vi "Ping Address.vi"(8 "error in (no error)":errorcluster, 9 "Number of pings(4)":i32=4, 10 "IP Address(loopback=127.0.0.1)":string="127.0.0.1", 11 "object in":refnum<class "Ghetto_ping.lvclass">) -> (0 "error out":errorcluster, 1 "Valid network address?":bool, 2 "Ping output":string, 3 "object out":refnum<class "Ghetto_ping.lvclass">)   [LabVIEW 2013, in "Ghetto_ping.lvclass"]
uses:
  Ghetto_ping.lvclass
panel:
  # "I AM REENTRANT"
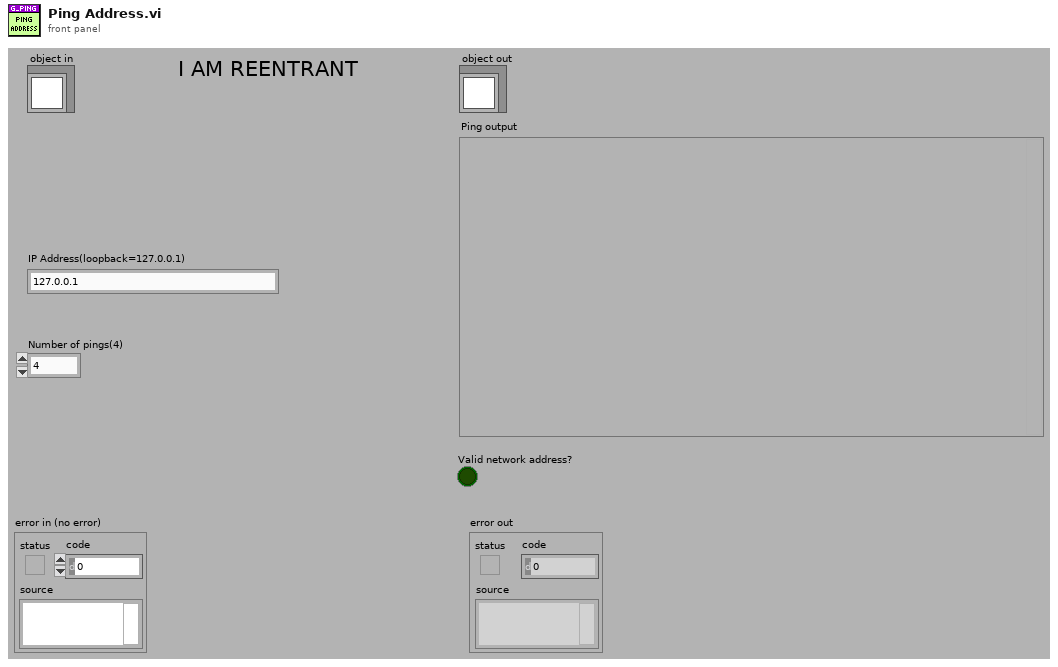
[diagram p1: front panel]
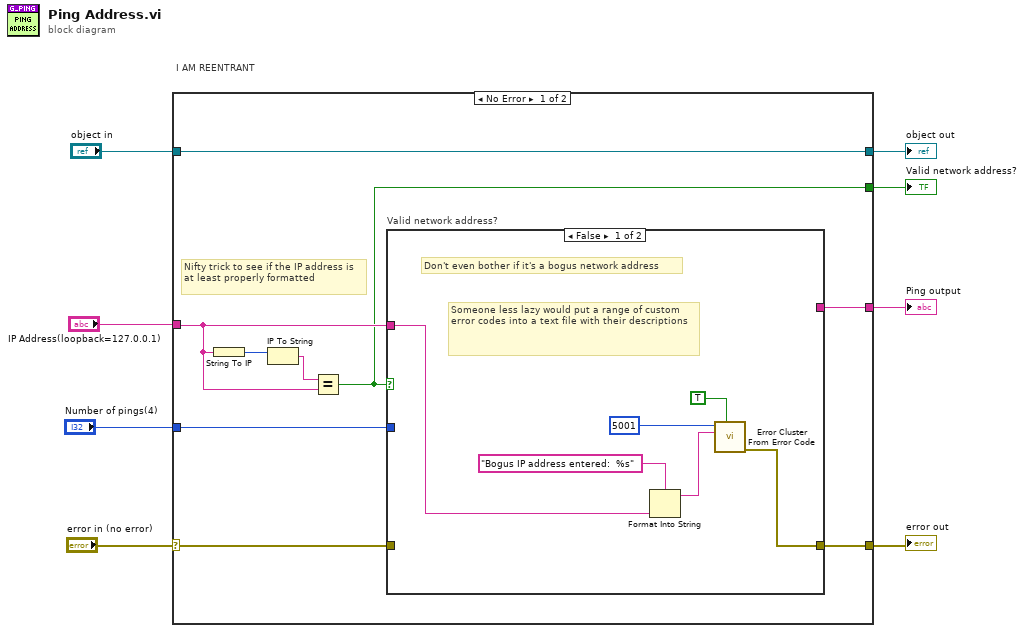
[diagram p0: block diagram]
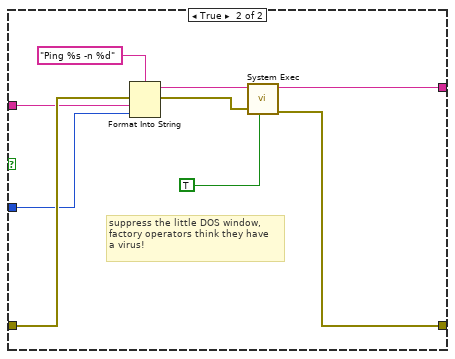
[diagram p2: hidden frame]
diagram:
  # "I AM REENTRANT"
  n1 = case shown="No Error" "error in (no error)" {
    selector: "error in (no error)" -> [w16 w34]
    tunnel: [w15 w34] -> w7
    tunnel: [w17 w33] -> w5
    tunnel: "object in" -> [w17 w33]
    tunnel: "IP Address(loopback=127.0.0.1)" -> [w10 _]
    tunnel: [w14 _] -> w3
    tunnel: "Number of pings(4)" -> [w13 _]
    tunnel: [w9 _] -> w1
    frame No Error {
      # "Nifty trick to see if the IP address is at least properly formatted"
      n2 = String To IP(1:w10) -> (0:w12:u32)
      n3 = IP To String(2:w12) -> (0:w11:string)  [unwired: 1 in]
      n4 = Equal?(x=w11, y=w10) -> (x = y?=w9:bool)
      n5 = case "Valid network address?" shown="False" w9 {
        tunnel: w16 -> [_ w28]
        tunnel: [w18 w27] -> w15
        tunnel: [_ w26] -> w14
        tunnel: w13 -> [_ w25]
        tunnel: w10 -> [w21 w24]
        frame False {
          # "Someone less lazy would put a range of custom error codes into a text file with their descriptions"
          # "Don't even bother if it's a bogus network address"
          n6 = Format Into String(format string="Bogus IP address entered:  %s", w21) -> (resulting string=w20:string)  [unwired: 2 in, 1 out]
          n7 = call <vilib>:"Error Cluster From Error Code.vi"("show call chain? (False)"=TRUE, "error message (\"\")"=w20, "error code (0)"=5001) -> ("error out"=w18:errorcluster)  [unwired: 6 in]
        }
        frame True {
          # "suppress the little DOS window,\nfactory operators think they have\na virus!"
          n8 = Format Into String(format string="Ping %s -n %d", error in=w28, w24, w25) -> (resulting string=w31:string, error out=w30:errorcluster)  [unwired: 1 in]
          n9 = call <vilib>:"System Exec.vi"("run minimized? (F)"=TRUE, "error in (no error)"=w30, "command line"=w31) -> ("error out"=w27:errorcluster, "standard output"=w26:string)  [unwired: 5 in, 2 out]
        }
      }
    }
    frame Error {
    }
  }
  "error out" <- w7
  "object out" <- w5
  "Ping output" <- w3
  "Valid network address?" <- w1
